vi "RunQDC.vi"() -> ()   [LabVIEW 2014]
uses:
  Program Files (x86)/CAEN/Comm/labview/CAENComm.lvlib
panel:
  out "Decode time":dbl
  in  "Low Range threshold":u16=1
  in  "High range threshold":u16=32
  out "Waveform Graph 3":u16[](graph)
  in  "stop":bool
  in  "Channel for hist":u8
  out "Results":T1(array[cluster]) {"GeoAddr" format="%.0x"}
  out "Error Read Value":u32 format="%.0x"
  out "Device was open?":bool
  out "error out":errorcluster
  in  "Count only accepted trigs?\n(else all trigs)":bool
  in  "# of events before transfer (max 32)":u16=32 min=1 max=32
  in  "IRQ Lvl":u16=1 format="%x"
  in  "CBLT Addr":u16=240 format="%x"
  in  "Geo Addr":u16=4 format="%x"
  in  "VME module Base Address":u32=4026793984 format="%x"
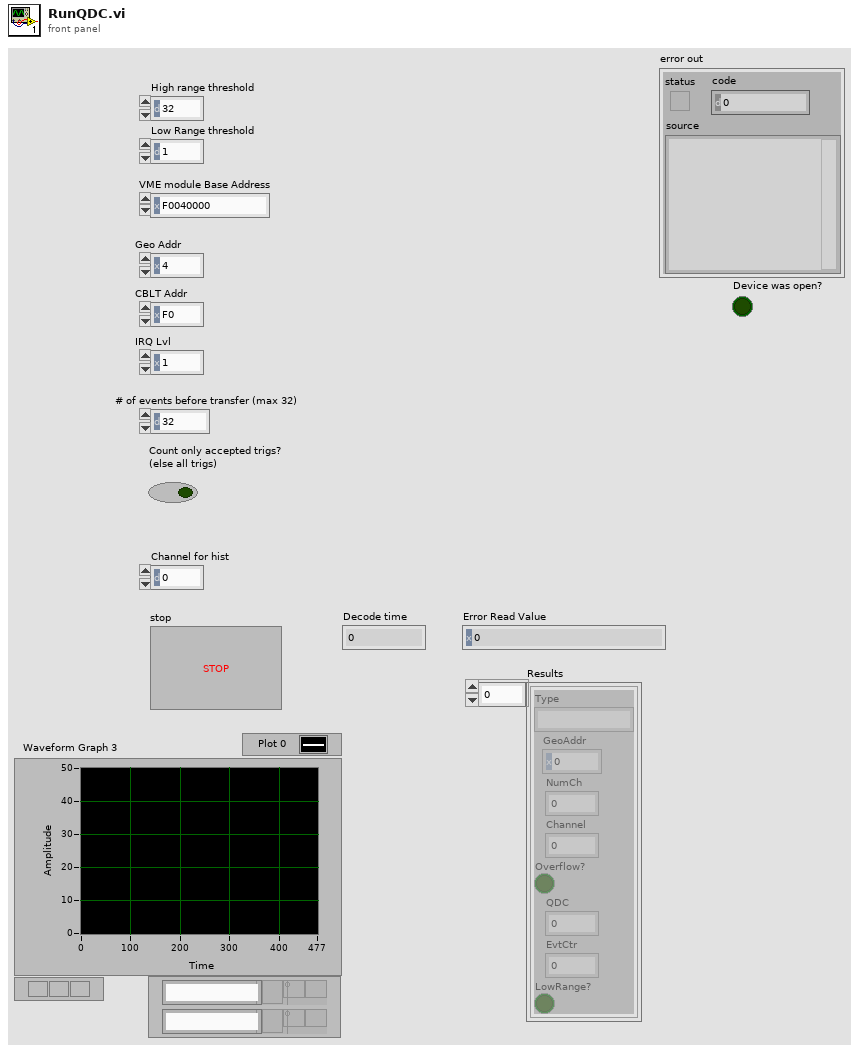
[diagram p1: front panel]
types:
  T1 = cluster{"Type":string, "GeoAddr":u8, "NumCh":u8, "Channel":u8, "Overflow?":bool, "QDC":u16, "EvtCtr":u32, "LowRange?":bool}[]
  T2 = cluster{"Type":string, "GeoAddr":u8, "NumCh":u8, "Channel":u8, "Overflow?":bool, "QDC":u16, "EvtCtr":u32, "LowRange?":bool}
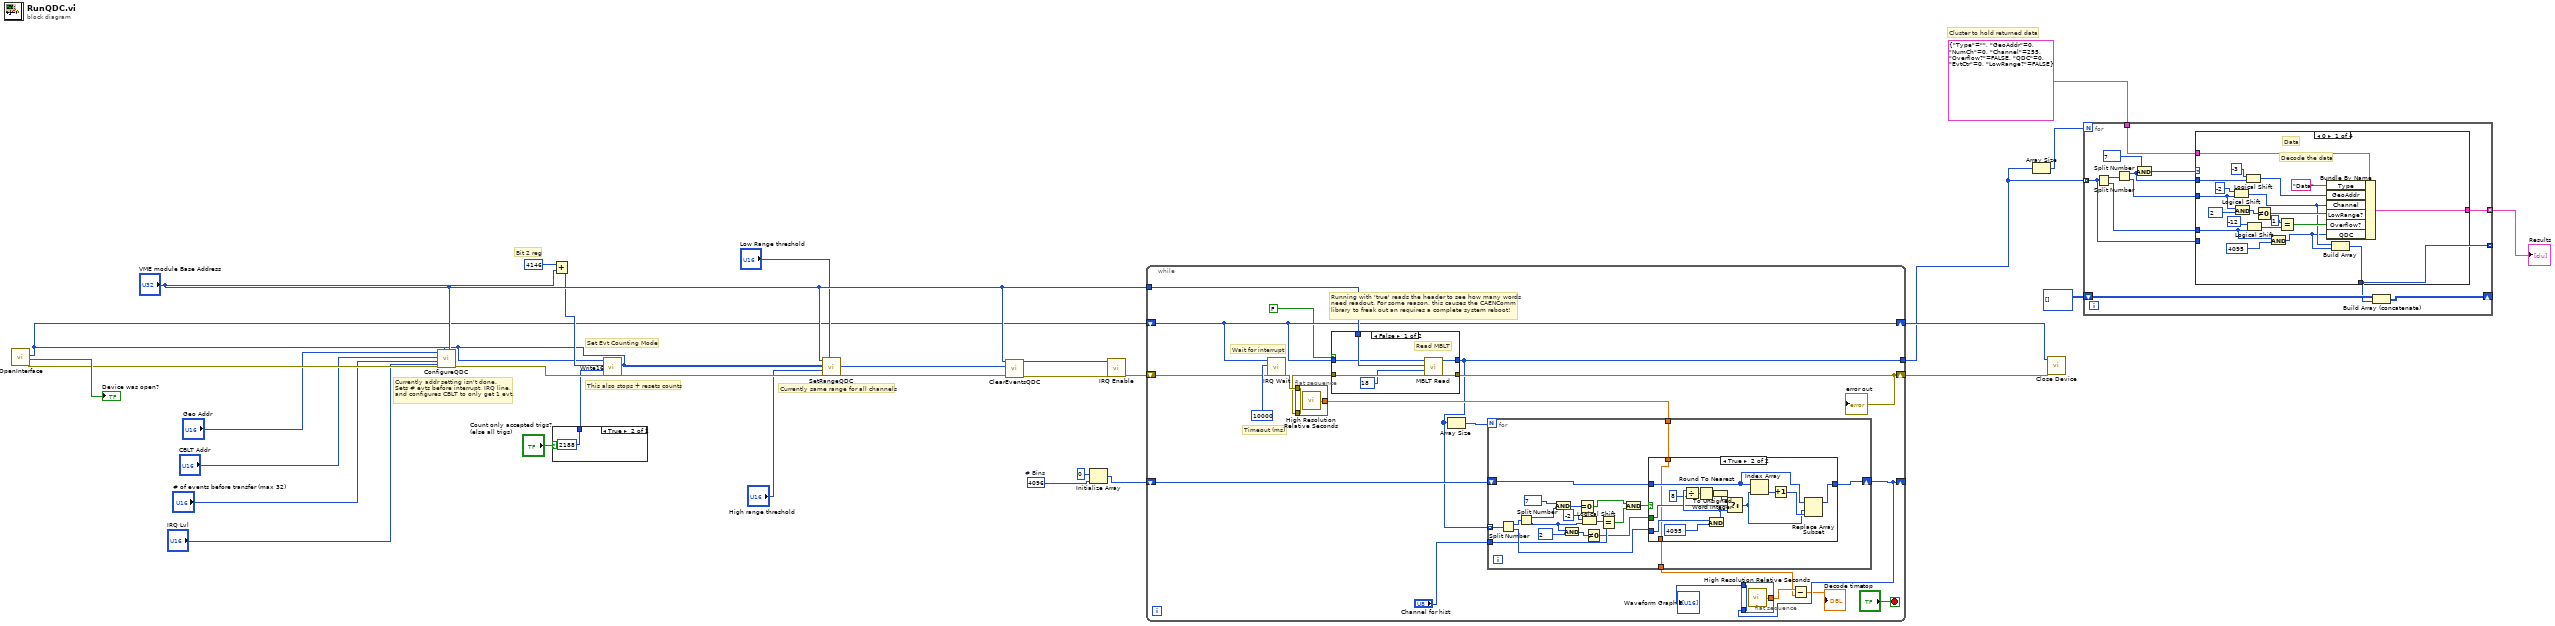
[diagram p0: block diagram]
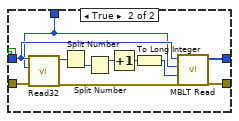
[diagram p2: hidden frame]
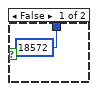
[diagram p4: hidden frame]
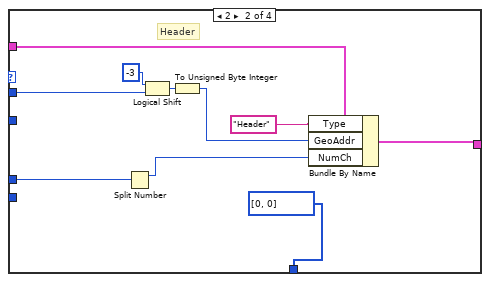
[diagram p5: hidden frame]
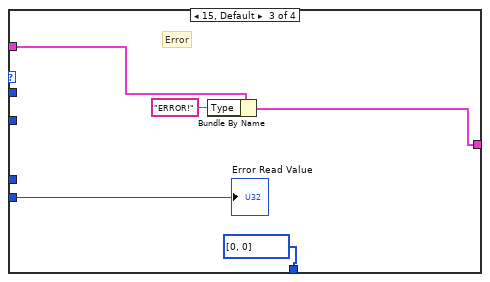
[diagram p6: hidden frame]
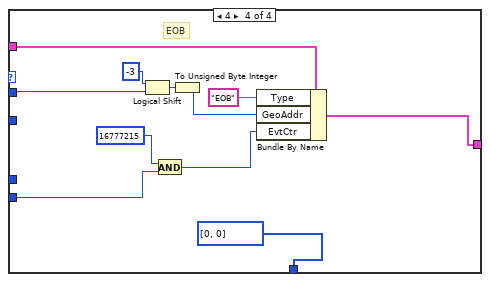
[diagram p7: hidden frame]
diagram:
  w10 = u16 4096  # # Bins
  # "Decode the data"
  # "Currently same range for all channels"
  # "Currently addr setting isn't done.\nSets # evts before interrupt, IRQ line,\nand configures CBLT to only get 1 evt."
  # "This also stops + resets counts"
  # "Bit 2 reg"
  # "Set Evt Counting Mode"
  # "Cluster to hold returned data"
  n1 = call "OpenInterface.vi"() -> ("error out"=w22:errorcluster, "specific error cleared?"=→"Device was open?":bool, "handle"=w5:i32)  [unwired: 9 in]
  n2 = call "ConfigureQDC.vi"("VME module Base Address"="VME module Base Address", "IRQ Lvl"="IRQ Lvl", "handle"=w5, "error in (no error)"=w22, "# of events before transfer (max 32)"="# of events before transfer (max 32)", "CBLT Addr"="CBLT Addr", "Geo Addr"="Geo Addr") -> ("error out"=w19:errorcluster)  [unwired: 4 in]
  n3 = case shown="True" "Count only accepted trigs?\n(else all trigs)" {
    tunnel: [18572 2188] -> w16
    frame False {
    }
    frame True {
    }
  }
  n4 = Add(x=u32 4146, y="VME module Base Address") -> (x+y=w13:u32)
  n5 = call "Write16.vi"("error in (no error)"=w19, "Data"=w16, "Address"=w13, "handle"=w5) -> ("error out"=w15:errorcluster)  [unwired: 7 in]
  n6 = call "SetRangeQDC.vi"("Low Range threshold"="Low Range threshold", "error in (no error)"=w15, "High range threshold"="High range threshold", "handle"=w5, "VME module Base Address"="VME module Base Address") -> ("error out"=w14:errorcluster)  [unwired: 6 in]
  n7 = call "ClearEventsQDC.vi"("error in (no error)"=w14, "handle"=w5, "VME module Base Address"="VME module Base Address") -> ("error out"=w3:errorcluster, "handle out"=w2:i32)  [unwired: 6 in, 1 out]
  n8 = Initialize Array(u16 0 ("element"), w10) -> (w12:u16[])
  n9 = call "IRQ Enable.vi"("error in (no error)"=w3, "handle"=w2) -> ("error out"=w1:errorcluster)  [unwired: 9 in]
  n10 = while {
    tunnel: "VME module Base Address" -> [w51]
    tunnel: [w35] -> w4
    shift-right: [w47] -> w29
    shift-left: w1 -> [w37]
    shift-right: [w38] -> w30
    shift-left: w5 -> [w38]
    shift-right: [w45] -> _
    shift-left: w12 -> [w50]
    stop <- "stop" stop-if-true
    # "Running with 'true' reads the header to see how many words\nneed readout. For some reason, this causes the CAENComm\nlibrary to freak out an requires a complete system reboot!"
    # "Wait for interrupt"
    # "Timeout (ms)"
    n11 = call "IRQ Wait.vi"("error in (no error)"=w37, "Timeout"=u32 10000, "handle"=w38) -> ("error out"=w34:errorcluster)  [unwired: 8 in]
    n12 = flat-sequence {
      tunnel: [w70] -> w33
      tunnel: w34 -> [w70]
      tunnel: [w69] -> w39
      frame #0 {
        n13 = call <vilib>:"High Resolution Relative Seconds.vi"() -> ("relative seconds"=w69:dbl)
      }
    }
    n14 = case shown="False" FALSE ("Readahead?") {
      tunnel: w33 -> [w57 w66]
      tunnel: w51 -> [w56 w60]
      tunnel: [w55 w68] -> w35
      tunnel: [w54 w67] -> w47
      tunnel: w38 -> [w52 w61]
      frame False {
        # "Read MBLT"
        n15 = call "MBLT Read.vi"("error in (no error)"=w57, "BltSize"=18, "Address"=w56, "handle"=w52) -> ("error out"=w54:errorcluster, "Buff"=w55:u32[])  [unwired: 5 in, 1 out]
      }
      frame True {
        n16 = call "Read32.vi"("error in (no error)"=w66, "Address"=w60, "handle"=w61) -> ("error out"=w64:errorcluster, "Data"=w65:u32)  [unwired: 7 in]
        n17 = Split Number(x=w65) -> (lo(x)=w63:u16)  [unwired: 1 out]
        n18 = Split Number(x=w63) -> (hi(x)=w62:u8)  [unwired: 1 out]
        n19 = Increment(x=w62) -> (x+1=w59:u8)
        n20 = To Long Integer(number=w59) -> (32bit integer=w58:i32)
        n21 = call "MBLT Read.vi"("error in (no error)"=w64, "BltSize"=w58, "Address"=w60, "handle"=w61) -> ("error out"=w67:errorcluster, "Buff"=w68:u32[])  [unwired: 5 in, 1 out]
      }
    }
    "error out" <- w47
    n22 = Array Size(array=w35) -> (size(s)=w40:i32)
    n23 = for {
      N: w40 -> [_]
      tunnel: w35 -> [w90] mode=indexing
      shift-right: [w78] -> w45
      shift-left: w50 -> [w79]
      tunnel: "Channel for hist" -> [w77]
      tunnel: w39 -> [w72]
      tunnel: [w71] -> w42
      n24 = Split Number(x=w90) -> (hi(x)=w89:u16, lo(x)=w86:u16)
      n25 = Split Number(x=w89) -> (hi(x)=w84:u8, lo(x)=w74:u8)
      n26 = And(x=u8 7, y=w84) -> (x .and. y?=w87:u8)
      n27 = And(x=w74, y=u8 2) -> (x .and. y?=w75:u8)
      n28 = Equal To 0?(x=w87) -> (x = 0?=w81:bool)
      n29 = Logical Shift(y=i16 -2, x=w74) -> (x << y=w83:u8)
      n30 = Not Equal To 0?(x=w75) -> (x != 0?=w73:bool)
      n31 = Equal?(x=w83, y=w77) -> (x = y?=w80:bool)
      n32 = And(x=w81, y=w80) -> (x .and. y?=w82:bool)
      n33 = case shown="True" w82 {
        tunnel: w86 -> [_ w105]
        tunnel: w79 -> [w92 w103]
        tunnel: [w92 w101] -> w78
        tunnel: w73 -> [_ w96]
        tunnel: w72 -> [w91 w93]
        tunnel: [w91 w93] -> w71
        frame False {
        }
        frame True {
          n34 = And(x=w105, y=u16 4095) -> (x .and. y?=w99:u16)
          n35 = Divide(x=w99, y=u16 8) -> (x/y=w100:dbl)
          n36 = Round To Nearest(number=w100) -> (nearest integer value=w95:dbl)
          n37 = To Unsigned Word Integer(number=w95) -> (unsigned 16bit integer=w94:u16)
          n38 = Select(t=w94, s=w96, f=w99) -> (s? t:f=w97:u16)
          n39 = Index Array(array=w103, index=w97) -> (element=w104:u16)
          n40 = Increment(x=w104) -> (x+1=w102:u16)
          n41 = Replace Array Subset(array=w103, new element=w102, index=w97) -> (w101:u16[])
        }
      }
    }
    n42 = flat-sequence {
      tunnel: w45 -> [w108]
      tunnel: [w108] -> w44
      tunnel: [w107] -> w43
      frame #0 {
        n43 = call <vilib>:"High Resolution Relative Seconds.vi"() -> ("relative seconds"=w107:dbl)
      }
    }
    n44 = Subtract(x=w43, y=w42) -> (x-y=→"Decode time":dbl)
    "Waveform Graph 3" <- w44
  }
  n45 = Array Size(array=w4) -> (size(s)=w26:i32)
  n46 = call "Close Device.vi"("error in (no error)"=w29, "handle"=w30) -> ()  [unwired: 9 in, 1 out]
  n47 = for {
    N: w26 -> [_]
    tunnel: w4 -> [w114] mode=indexing
    tunnel: T2 {"Type"="", "GeoAddr"=0, "NumCh"=0, "Channel"=255, "Overflow?"=FALSE, "QDC"=0, "EvtCtr"=0, "LowRange?"=FALSE} -> [w117]
    tunnel: [w112] -> w24 mode=indexing
    tunnel: [w110] -> _ mode=indexing
    shift-right: [w109] -> _
    shift-left: u32[][] [] -> [w111]
    n48 = Split Number(x=w114) -> (hi(x)=w120:u16, lo(x)=w115:u16)
    n49 = Split Number(x=w120) -> (hi(x)=w116:u8, lo(x)=w113:u8)
    n50 = And(x=u8 7, y=w116) -> (x .and. y?=w118:u8)
    n51 = case shown="0" w118 {
      tunnel: w117 -> [w140 w146 w155 w166]
      tunnel: w116 -> [w137 w150 _ w162]
      tunnel: w115 -> [w129 w147 _ _]
      tunnel: w114 -> [_ _ w153 w160]
      tunnel: w113 -> [w135 _ _ _]
      tunnel: [w127 w142 w152 w157] -> w112
      tunnel: [w121 u32[] [0, 0] ("Buff") u32[] [0, 0] ("Buff") u32[] [0, 0] ("Buff")] -> w110
      frame 0 {
        # "Data"
        n52 = Logical Shift(y=i16 -2, x=w135) -> (x << y=w123:u8)
        n53 = And(x=w135, y=u8 2) -> (x .and. y?=w133:u8)
        n54 = Logical Shift(y=i16 -3, x=w137) -> (x << y=w131:u8)
        n55 = Logical Shift(y=i16 -12, x=w129) -> (x << y=w126:u16)
        n56 = Not Equal To 0?(x=w133) -> (x != 0?=w132:bool)
        n57 = And(x=w129, y=u16 4095) -> (x .and. y?=w122:u16)
        n58 = Equal?(x=u16 1, y=w126) -> (x = y?=w124:bool)
        n59 = Bundle By Name(cluster=w140, "Type"="Data", "GeoAddr"=w131, "Channel"=w123, "LowRange?"=w132, "Overflow?"=w124, "QDC"=w122) -> (w127:T2)
        n60 = Build Array(w123, w122) -> (w121:u16[])
      }
      frame 2 {
        # "Header"
        n61 = Split Number(x=w147) -> (hi(x)=w143:u8)  [unwired: 1 out]
        n62 = Logical Shift(y=i16 -3, x=w150) -> (x << y=w148:u8)
        n63 = To Unsigned Byte Integer(number=w148) -> (unsigned 8bit integer=w144:u8)
        n64 = Bundle By Name(cluster=w146, "Type"="Header", "GeoAddr"=w144, "NumCh"=w143) -> (w142:T2)
      }
      frame 15, Default {
        # "Error"
        n65 = Bundle By Name(cluster=w155, "Type"="ERROR!") -> (w152:T2)
        "Error Read Value" <- w153
      }
      frame 4 {
        # "EOB"
        n66 = Logical Shift(y=i16 -3, x=w162) -> (x << y=w164:u8)
        n67 = And(x=u32 16777215, y=w160) -> (x .and. y?=w158:u32)
        n68 = To Unsigned Byte Integer(number=w164) -> (unsigned 8bit integer=w161:u8)
        n69 = Bundle By Name(cluster=w166, "Type"="EOB", "GeoAddr"=w161, "EvtCtr"=w158) -> (w157:T2)
      }
    }
    n70 = Build Array (concatenate)(w111, w110) -> (w109:u32[][])
  }
  "Results" <- w24
